vi "Table_AssertRowValue_Tests.vi"(8 "error in":errorcluster) -> (0 "error out":errorcluster)   [LabVIEW 2016, in "DronaTest.lvlib"]
uses:
  DronaTest.lvlib
  APIs/Stimulus/ControlValue/SetValueAuto.vi
  APIs/Assert/AssertControlValue/Controls/Table/AssertRowValue.vi
  <vilib>/addons/_JKI Toolkits/Caraya/classes/Assert/Assert Equal Value_Variant.vi
  <vilib>/addons/_JKI Toolkits/Caraya/classes/Test/Test.lvclass
  <vilib>/SLL Toolkit/SLL Debug/SLL Debug.lvlib
  Drona.lvlib
  <vilib>/addons/_JKI Toolkits/Caraya/classes/Assert/Assert.lvclass
  APIs/Get/GetControlRef/GetControlRef.lvlib
  APIs/Stimulus/ControlValue/ControlValue.lvlib
  APIs/Assert/AssertControlValue/Controls/Table/AssertTable.lvlib
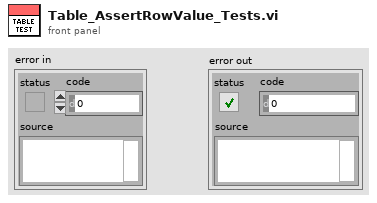
[diagram p1: front panel]
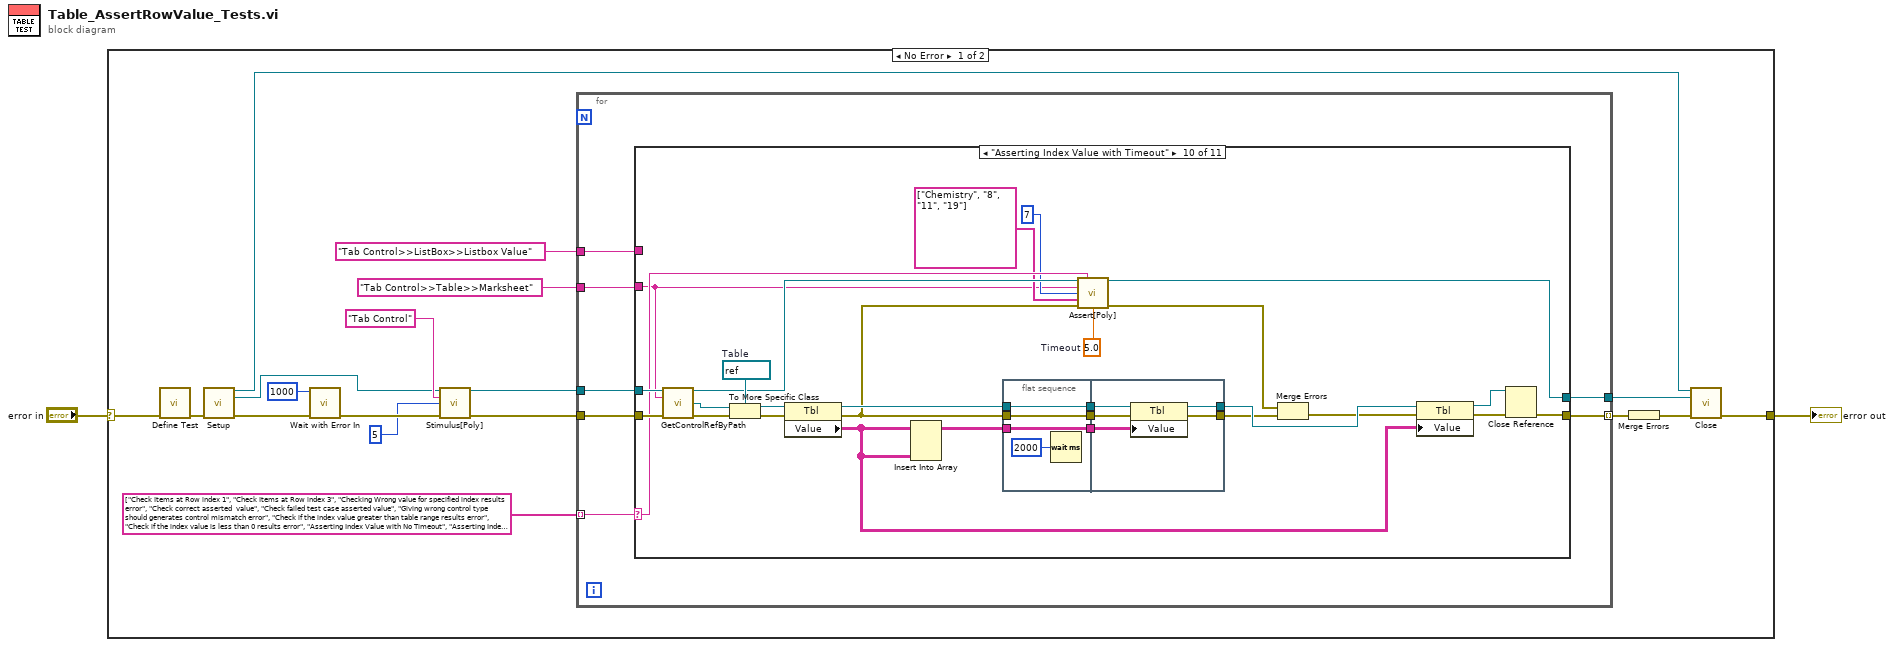
[diagram p0: block diagram]
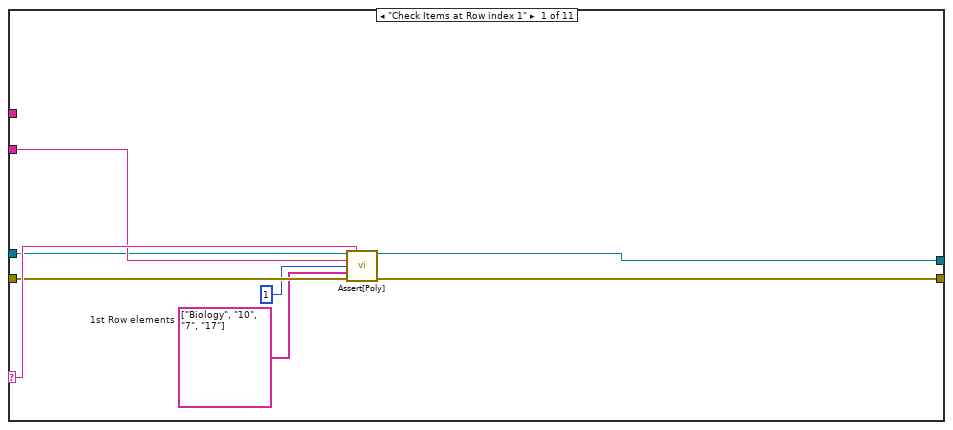
[diagram p2: hidden frame]
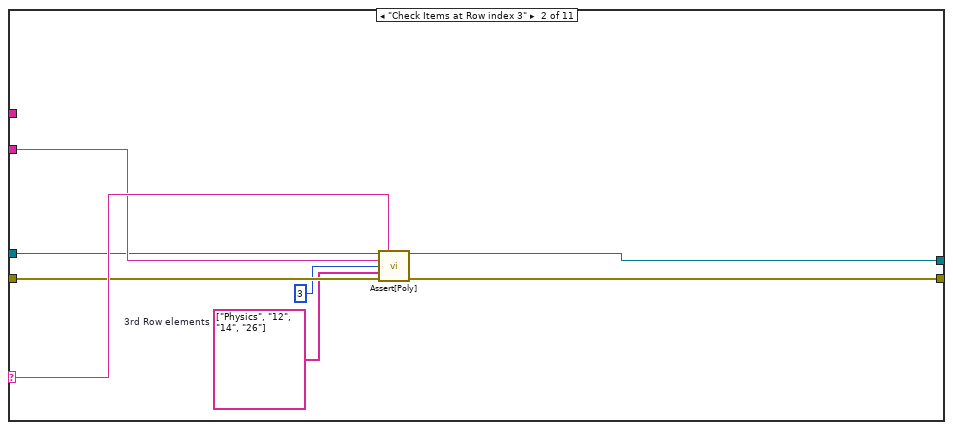
[diagram p3: hidden frame]
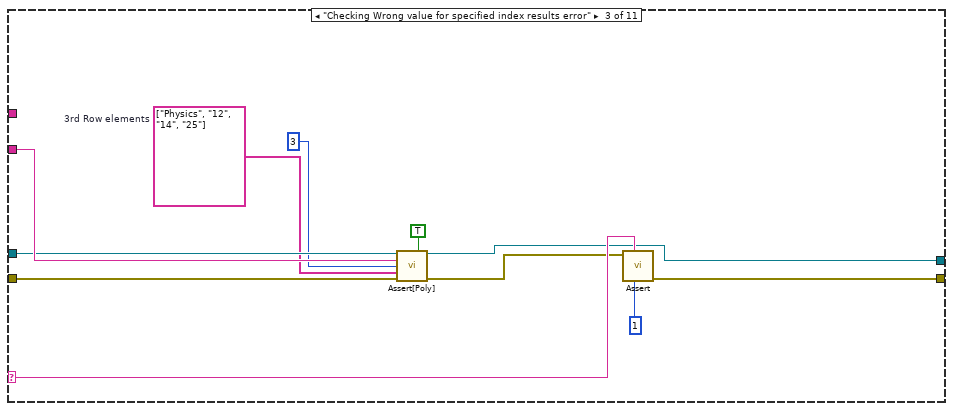
[diagram p4: hidden frame]
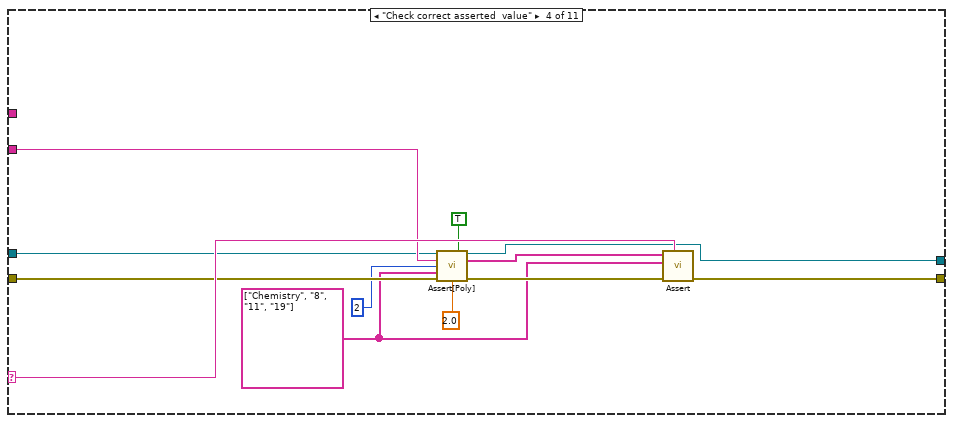
[diagram p5: hidden frame]
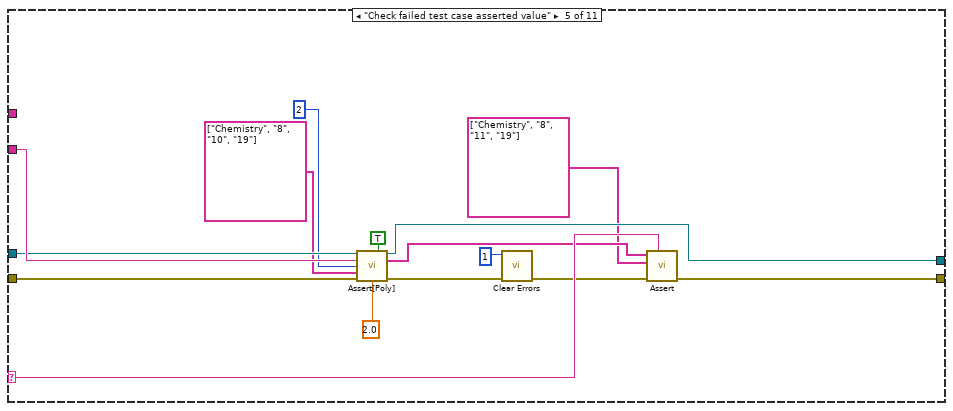
[diagram p6: hidden frame]
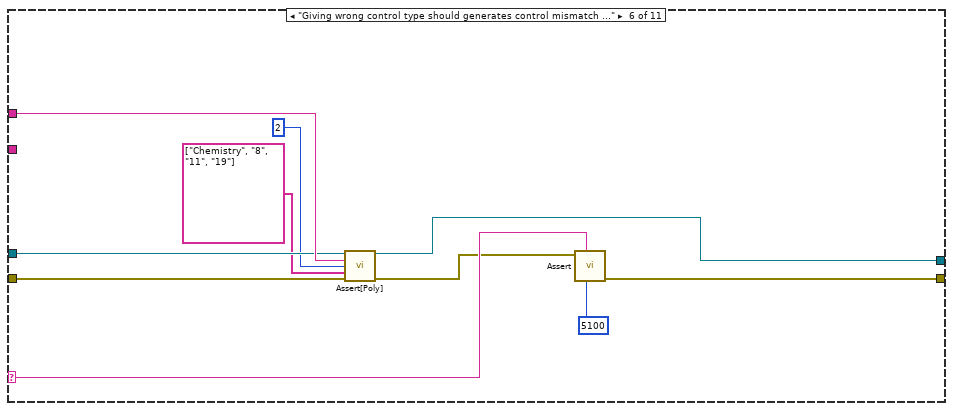
[diagram p7: hidden frame]
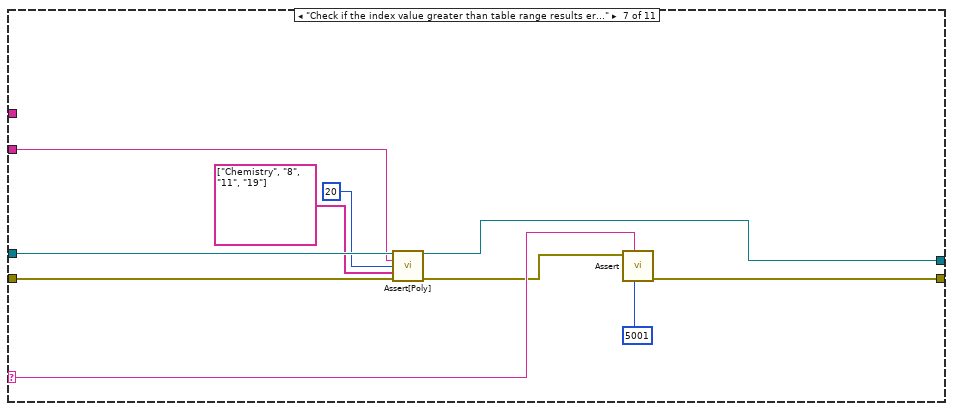
[diagram p8: hidden frame]
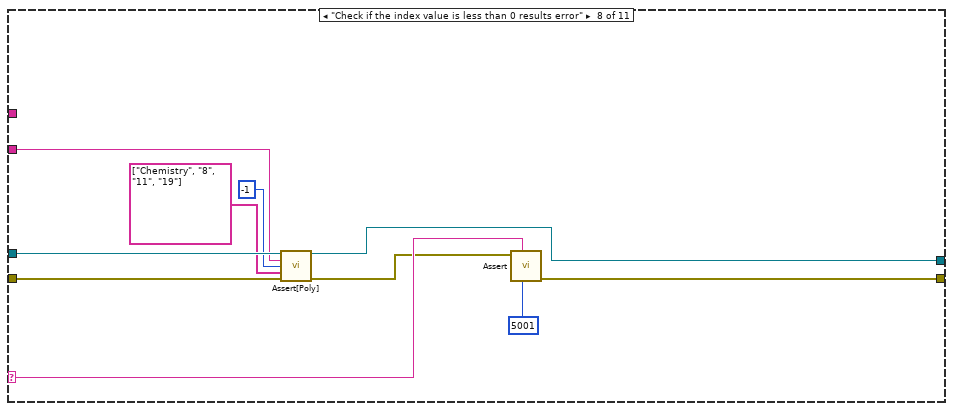
[diagram p9: hidden frame]
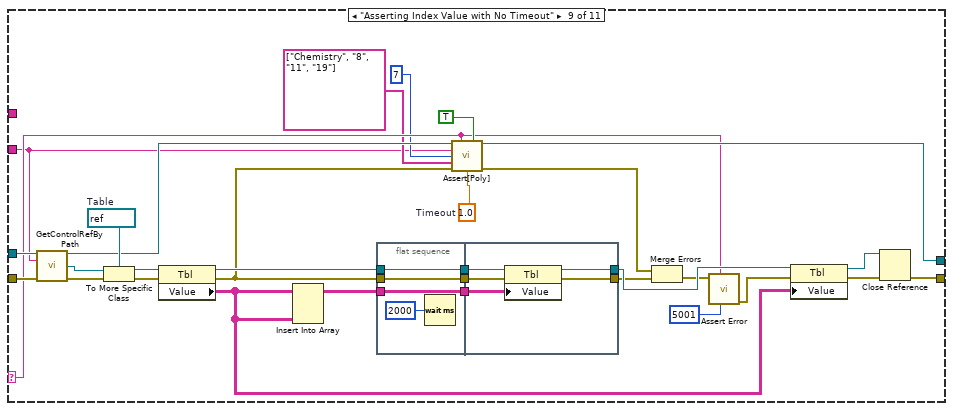
[diagram p10: hidden frame]
diagram:
  n1 = case shown="No Error" "error in" {
    selector: "error in" -> [w20 w191]
    tunnel: [w3 w191] -> w1
    frame No Error {
      n2 = call <vilib>:"Define Test.vi"("error in (no error)"=w20) -> ("error out"=w9:errorcluster)  [unwired: 9 in, 1 out]
      n3 = call "Setup.vi"("error in"=w9) -> ("Application Ref"=w5:refnum<vi>, "VI Reference Out"=w7:refnum<vi>, "error out"=w8:errorcluster)  [unwired: 12 in]
      n4 = call <vilib>:"Wait with Error In.vi"("error in (no error)"=w8, "milliseconds to wait"=u32 1000) -> ("error out"=w18:errorcluster)  [unwired: 9 in]
      n5 = call-poly "Stimulus[Poly].vi"("VI Reference In"=w7, "Control Path"="Tab Control", "Value (Signaling)"=5, "error in"=w18) -> ("VI Reference Out"=w14:refnum<vi>, "error out"=w17:errorcluster)  [unwired: 10 in]
      n6 = for {
        tunnel: w14 -> [w23]
        tunnel: "Tab Control>>Table>>Marksheet" ("Control Path") -> [w21]
        tunnel: "Tab Control>>ListBox>>Listbox Value" ("Control Path") -> [w22]
        tunnel: string[] ["Check Items at Row index 1", "Check Items at Row index 3", "Checking Wrong value for specified index results error", "Check correct asserted  value", "Check failed test case asserted value", "Giving wrong control type should generates control mismatch error", "Check if the index value greater than table range results error", "Check if the index value is less than 0 results error", "Asserting Index Value with No Timeout", "Asserting Index Value with Timeout"] -> [w27] mode=indexing
        tunnel: [w25] -> w4
        tunnel: w17 -> [w24]
        tunnel: [w26] -> w10 mode=indexing
        n7 = case shown="\"Asserting Index Value with Timeout\"" w27 {
          selector: w27 -> [w33 w41 w53 w65 w80 w90 w100 w110 w117 w169 _]
          tunnel: w24 -> [w31 w39 w47 w61 w76 w85 w96 w106 w142 w179 w190]
          tunnel: w23 -> [w30 w38 w46 w60 w75 w84 w95 w105 w140 w177 w189]
          tunnel: w21 -> [w32 w40 w51 w64 w79 _ w94 w104 w112 w152 _]
          tunnel: w22 -> [_ _ _ _ _ w87 _ _ _ _ _]
          tunnel: [w35 w43 w54 w66 w81 w91 w101 w111 w129 w165 w190] -> w26
          tunnel: [w34 w42 w50 w63 w78 w86 w97 w107 w133 w170 w189] -> w25
          frame "Check Items at Row index 1" {
            w28 = string[] ["Biology", "10", "7", "17"]  # 1st Row elements
            n8 = call-poly "Assert[Poly].vi"("VI Reference In"=w30, "Test Label"=w33, "Control Path"=w32, "Row Index"=1 ("Item Index"), "Item Value"=w28, "Error In"=w31) -> ("VI Reference Out"=w34:refnum<vi>, "Error Out"=w35:errorcluster)  [unwired: 7 in, 1 out]
          }
          frame "Check Items at Row index 3" {
            w36 = string[] ["Physics", "12", "14", "26"]  # 3rd Row elements
            n9 = call-poly "Assert[Poly].vi"("VI Reference In"=w38, "Test Label"=w41, "Control Path"=w40, "Row Index"=3 ("Item Index"), "Item Value"=w36, "Error In"=w39) -> ("VI Reference Out"=w42:refnum<vi>, "Error Out"=w43:errorcluster)  [unwired: 7 in, 1 out]
          }
          frame "Checking Wrong value for specified index results error" {
            w44 = string[] ["Physics", "12", "14", "25"]  # 3rd Row elements
            n10 = call-poly "Assert[Poly].vi"("VI Reference In"=w46, "Assert Only? (F)"=TRUE, "Control Path"=w51, "Row Index"=3 ("Item Index"), "Item Value"=w44, "Error In"=w47) -> ("VI Reference Out"=w50:refnum<vi>, "Error Out"=w49:errorcluster)  [unwired: 7 in, 1 out]
            n11 = call-poly <vilib>:"Assert.vi"("error code (1)"=1, "Label"=w53, "Error?"=w49) -> ("error out"=w54:errorcluster)  [unwired: 7 in, 1 out]
          }
          frame "Check correct asserted  value" {
            w55 = string[] ["Chemistry", "8", "11", "19"] ("Row Value")
            n12 = call-poly "Assert[Poly].vi"("VI Reference In"=w60, "Assert Only? (F)"=TRUE, "Control Path"=w64, "Row Index"=2 ("Item Index"), "Item Value"=w55, "Error In"=w61, "Timeout(5 sec)"=2.0) -> ("VI Reference Out"=w63:refnum<vi>, "Asserted Value"=w58:string[], "Error Out"=w59:errorcluster)  [unwired: 6 in]
            n13 = call-poly <vilib>:"Assert.vi"("Label"=w65, "error in (no error)"=w59, "Y"=w55, "X"=w58) -> ("error out"=w66:errorcluster)  [unwired: 6 in, 1 out]
          }
          frame "Check failed test case asserted value" {
            n14 = call-poly "Assert[Poly].vi"("VI Reference In"=w75, "Assert Only? (F)"=TRUE, "Control Path"=w79, "Row Index"=2 ("Item Index"), "Item Value"=string[] ["Chemistry", "8", "10", "19"] ("Row Value"), "Error In"=w76, "Timeout(5 sec)"=2.0) -> ("VI Reference Out"=w78:refnum<vi>, "Asserted Value"=w73:string[], "Error Out"=w74:errorcluster)  [unwired: 6 in]
            n15 = call <vilib>:"Clear Errors.vi"("error in (no error)"=w74, "specific error code to clear (0: all)"=1) -> ("error out"=w72:errorcluster)  [unwired: 4 in, 1 out]
            n16 = call-poly <vilib>:"Assert.vi"("Label"=w80, "error in (no error)"=w72, "Y"=string[] ["Chemistry", "8", "11", "19"] ("Row Value"), "X"=w73) -> ("error out"=w81:errorcluster)  [unwired: 6 in, 1 out]
          }
          frame "Giving wrong control type should generates control mismatch error" {
            n17 = call-poly "Assert[Poly].vi"("VI Reference In"=w84, "Control Path"=w87, "Row Index"=2 ("Item Index"), "Item Value"=string[] ["Chemistry", "8", "11", "19"] ("Row Value"), "Error In"=w85) -> ("VI Reference Out"=w86:refnum<vi>, "Error Out"=w88:errorcluster)  [unwired: 8 in, 1 out]
            n18 = call-poly <vilib>:"Assert.vi"("error code (1)"=5100, "Label"=w90, "Error?"=w88) -> ("error out"=w91:errorcluster)  [unwired: 7 in, 1 out]
          }
          frame "Check if the index value greater than table range results error" {
            n19 = call-poly "Assert[Poly].vi"("VI Reference In"=w95, "Control Path"=w94, "Row Index"=20 ("Item Index"), "Item Value"=string[] ["Chemistry", "8", "11", "19"] ("Row Value"), "Error In"=w96) -> ("VI Reference Out"=w97:refnum<vi>, "Error Out"=w98:errorcluster)  [unwired: 8 in, 1 out]
            n20 = call-poly <vilib>:"Assert.vi"("error code (1)"=5001, "Label"=w100, "Error?"=w98) -> ("error out"=w101:errorcluster)  [unwired: 7 in, 1 out]
          }
          frame "Check if the index value is less than 0 results error" {
            n21 = call-poly "Assert[Poly].vi"("VI Reference In"=w105, "Control Path"=w104, "Row Index"=-1 ("Item Index"), "Item Value"=string[] ["Chemistry", "8", "11", "19"] ("Row Value"), "Error In"=w106) -> ("VI Reference Out"=w107:refnum<vi>, "Error Out"=w108:errorcluster)  [unwired: 8 in, 1 out]
            n22 = call-poly <vilib>:"Assert.vi"("error code (1)"=5001, "Label"=w110, "Error?"=w108) -> ("error out"=w111:errorcluster)  [unwired: 7 in, 1 out]
          }
          frame "Asserting Index Value with No Timeout" {
            w126 = 1.0  # Timeout
            w137 = refnum<vi> refnum  # Table
            n23 = call "GetControlRefByPath.vi"("VI Reference In"=w140, "Control Path"=w112, "error In"=w142) -> ("VI Reference Out"=w134:refnum<vi>, "Ctl Refnum"=w138:refnum<vi>, "error out"=w141:errorcluster)  [unwired: 10 in]
            n24 = To More Specific Class(target class=w137, reference=w138, error in=w141) -> (specific class reference=w136:refnum<vi>, error out=w139:errorcluster)
            n25 = property class="Tbl"(reference=w136, error in=w139) -> (reference out=w132:refnum<vi>, error out=w125:errorcluster, "Value"=w115:string[][])
            n26 = Insert Into Array(array=w115, new element=w115) -> (w135:string[][])  [unwired: 2 in]
            n27 = flat-sequence {
              tunnel: w125 -> [w144]
              tunnel: w132 -> [w145]
              tunnel: w135 -> [w146]
              tunnel: [w146] -> w123
              tunnel: [w145] -> w122
              tunnel: [w144] -> w121
              tunnel: [w149] -> w128
              tunnel: [w147] -> w124
              tunnel: w123 -> [w151]
              tunnel: w122 -> [w150]
              tunnel: w121 -> [w148]
              frame #0 {
                n28 = Wait (ms)(milliseconds to wait=u32 2000) -> ()  [unwired: 1 out]
              }
              frame #1 {
                n29 = property class="Tbl"(reference=w150, error in=w148, "Value"=w151) -> (reference out=w149:refnum<vi>, error out=w147:errorcluster)
              }
            }
            n30 = call-poly "Assert[Poly].vi"("VI Reference In"=w134, "Test Label"=w117, "Assert Only? (F)"=TRUE, "Control Path"=w112, "Row Index"=7, "Item Value"=string[] ["Chemistry", "8", "11", "19"] ("Row Value"), "Error In"=w125, "Timeout(5 sec)"=w126) -> ("VI Reference Out"=w133:refnum<vi>, "Error Out"=w131:errorcluster)  [unwired: 5 in, 1 out]
            n31 = Merge Errors(w131, w124) -> (w120:errorcluster)
            n32 = call <vilib>:"Assert Error.vi"("error code (1)"=5001, "Label"=w117, "Error?"=w120) -> ("error out"=w119:errorcluster)  [unwired: 7 in, 1 out]
            n33 = property class="Tbl"(reference=w128, error in=w119, "Value"=w115) -> (reference out=w127:refnum<vi>, error out=w130:errorcluster)
            n34 = Close Reference(reference=w127, error in (no error)=w130) -> (error out=w129:errorcluster)
          }
          frame "Asserting Index Value with Timeout" {
            w156 = 5.0  # Timeout
            w174 = refnum<vi> refnum  # Table
            n35 = call "GetControlRefByPath.vi"("VI Reference In"=w177, "Control Path"=w152, "error In"=w179) -> ("VI Reference Out"=w171:refnum<vi>, "Ctl Refnum"=w175:refnum<vi>, "error out"=w178:errorcluster)  [unwired: 10 in]
            n36 = To More Specific Class(target class=w174, reference=w175, error in=w178) -> (specific class reference=w173:refnum<vi>, error out=w176:errorcluster)
            n37 = property class="Tbl"(reference=w173, error in=w176) -> (reference out=w168:refnum<vi>, error out=w162:errorcluster, "Value"=w155:string[][])
            n38 = Insert Into Array(array=w155, new element=w155) -> (w172:string[][])  [unwired: 2 in]
            n39 = flat-sequence {
              tunnel: w162 -> [w181]
              tunnel: w168 -> [w182]
              tunnel: w172 -> [w183]
              tunnel: [w183] -> w159
              tunnel: [w182] -> w158
              tunnel: [w181] -> w157
              tunnel: [w186] -> w164
              tunnel: [w184] -> w160
              tunnel: w159 -> [w188]
              tunnel: w158 -> [w187]
              tunnel: w157 -> [w185]
              frame #0 {
                n40 = Wait (ms)(milliseconds to wait=u32 2000) -> ()  [unwired: 1 out]
              }
              frame #1 {
                n41 = property class="Tbl"(reference=w187, error in=w185, "Value"=w188) -> (reference out=w186:refnum<vi>, error out=w184:errorcluster)
              }
            }
            n42 = call-poly "Assert[Poly].vi"("VI Reference In"=w171, "Test Label"=w169, "Control Path"=w152, "Row Index"=7, "Item Value"=string[] ["Chemistry", "8", "11", "19"] ("Row Value"), "Error In"=w162, "Timeout(5 sec)"=w156) -> ("VI Reference Out"=w170:refnum<vi>, "Error Out"=w167:errorcluster)  [unwired: 6 in, 1 out]
            n43 = Merge Errors(w167, w160) -> (w161:errorcluster)
            n44 = property class="Tbl"(reference=w164, error in=w161, "Value"=w155) -> (reference out=w163:refnum<vi>, error out=w166:errorcluster)
            n45 = Close Reference(reference=w163, error in (no error)=w166) -> (error out=w165:errorcluster)
          }
          frame Default {
          }
        }
      }
      n46 = Merge Errors(w10) -> (w6:errorcluster)
      n47 = call "Close.vi"("Application Ref"=w5, "VI Reference"=w4, "error in"=w6) -> ("error out"=w3:errorcluster)  [unwired: 12 in]
    }
    frame Error {
    }
  }
  "error out" <- w1
